vi "QCP_Load.vi"   [LabVIEW 2016]
uses:
  <userlib>/836-libraries/System/QCP_V2/QCPSupportCode/QCP_GetDbl.vi
  <userlib>/836-libraries/System/QCP_V2/QCPSupportCode/QCP_GetDblArr.vi
types:
  T1 = typedef "QCP_RefNum.ctl" = cluster{"Data Value Refnum":refnum<data-value>, "semaphore":T2}
  T2 = typedef "Semaphore RefNum" = refnum<k1>
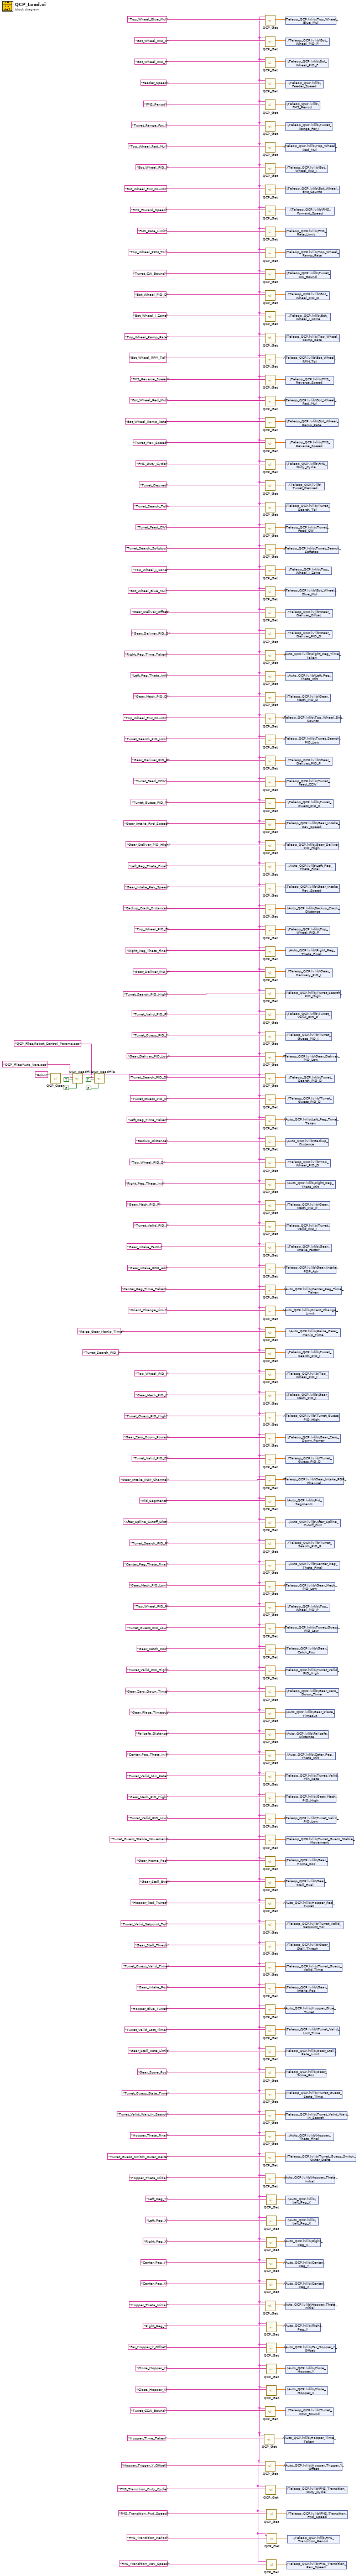
[diagram p0: block diagram]
diagram:
  n1 = call <userlib>:"QCP_Open.vi"("Name"="Robot") -> ("QCP_DevRef_Out"=w250:T1)  [unwired: 9 in, 1 out]
  n2 = call <userlib>:"QCP_ReadFile.vi"("Overrite Existing Data?"=FALSE ("Path Relative?"), "Path Relative?"=TRUE, "Path"="QCP_Files/Auto_Vars.qcp", "QCP_DevRef_In"=w250) -> ("QCP_DevRef_Out"=w245:T1)  [unwired: 6 in, 1 out]
  n3 = call <userlib>:"QCP_ReadFile.vi"("Overrite Existing Data?"=FALSE ("Path Relative?"), "Path Relative?"=TRUE, "Path"="QCP_Files/Robot_Control_Params.qcp", "QCP_DevRef_In"=w245) -> ("QCP_DevRef_Out"=w1:T1)  [unwired: 6 in, 1 out]
  n4 = call-poly <userlib>:"QCP_Get.vi"("Value Name"="Hopper_Time_Taken", "QCP_DevRef_In"=w1) -> ("Value"=w13:dbl)  [unwired: 7 in, 2 out]
  n5 = call-poly <userlib>:"QCP_Get.vi"("Value Name"="Top_Wheel_Blue_Mul", "QCP_DevRef_In"=w1) -> ("Value"=w75:dbl)  [unwired: 7 in, 2 out]
  n6 = call-poly <userlib>:"QCP_Get.vi"("Value Name"="Bot_Wheel_PID_P", "QCP_DevRef_In"=w1) -> ("Value"=w71:dbl)  [unwired: 7 in, 2 out]
  n7 = call-poly <userlib>:"QCP_Get.vi"("Value Name"="Bot_Wheel_PID_F", "QCP_DevRef_In"=w1) -> ("Value"=w70:dbl)  [unwired: 7 in, 2 out]
  n8 = call-poly <userlib>:"QCP_Get.vi"("Value Name"="Feeder_Speed", "QCP_DevRef_In"=w1) -> ("Value"=w102:dbl)  [unwired: 7 in, 2 out]
  n9 = call-poly <userlib>:"QCP_Get.vi"("Value Name"="FMS_Period", "QCP_DevRef_In"=w1) -> ("Value"=w25:dbl)  [unwired: 7 in, 2 out]
  n10 = call-poly <userlib>:"QCP_Get.vi"("Value Name"="Turret_Range_For_I", "QCP_DevRef_In"=w1) -> ("Value"=w17:dbl)  [unwired: 7 in, 2 out]
  n11 = call-poly <userlib>:"QCP_Get.vi"("Value Name"="Top_Wheel_Red_Mul", "QCP_DevRef_In"=w1) -> ("Value"=w76:dbl)  [unwired: 7 in, 2 out]
  n12 = call-poly <userlib>:"QCP_Get.vi"("Value Name"="Bot_Wheel_PID_I", "QCP_DevRef_In"=w1) -> ("Value"=w72:dbl)  [unwired: 7 in, 2 out]
  n13 = call-poly <userlib>:"QCP_Get.vi"("Value Name"="Bot_Wheel_Enc_Counts", "QCP_DevRef_In"=w1) -> ("Value"=w69:dbl)  [unwired: 7 in, 2 out]
  n14 = call-poly <userlib>:"QCP_Get.vi"("Value Name"="FMS_Foward_Speed", "QCP_DevRef_In"=w1) -> ("Value"=w101:dbl)  [unwired: 7 in, 2 out]
  n15 = call-poly <userlib>:"QCP_Get.vi"("Value Name"="FMS_Rate_Limit", "QCP_DevRef_In"=w1) -> ("Value"=w27:dbl)  [unwired: 7 in, 2 out]
  n16 = call-poly <userlib>:"QCP_Get.vi"("Value Name"="Top_Wheel_RPM_Tol", "QCP_DevRef_In"=w1) -> ("Value"=w77:dbl)  [unwired: 7 in, 2 out]
  n17 = call-poly <userlib>:"QCP_Get.vi"("Value Name"="Turret_CW_Bound", "QCP_DevRef_In"=w1) -> ("Value"=w24:dbl)  [unwired: 7 in, 2 out]
  n18 = call-poly <userlib>:"QCP_Get.vi"("Value Name"="Bot_Wheel_PID_D", "QCP_DevRef_In"=w1) -> ("Value"=w73:dbl)  [unwired: 7 in, 2 out]
  n19 = call-poly <userlib>:"QCP_Get.vi"("Value Name"="Bot_Wheel_I_Zone", "QCP_DevRef_In"=w1) -> ("Value"=w68:dbl)  [unwired: 7 in, 2 out]
  n20 = call-poly <userlib>:"QCP_Get.vi"("Value Name"="Top_Wheel_Ramp_Rate", "QCP_DevRef_In"=w1) -> ("Value"=w78:dbl)  [unwired: 7 in, 2 out]
  n21 = call-poly <userlib>:"QCP_Get.vi"("Value Name"="Bot_Wheel_RPM_Tol", "QCP_DevRef_In"=w1) -> ("Value"=w74:dbl)  [unwired: 7 in, 2 out]
  n22 = call-poly <userlib>:"QCP_Get.vi"("Value Name"="FMS_Reverse_Speed", "QCP_DevRef_In"=w1) -> ("Value"=w100:dbl)  [unwired: 7 in, 2 out]
  n23 = call-poly <userlib>:"QCP_Get.vi"("Value Name"="Bot_Wheel_Red_Mul", "QCP_DevRef_In"=w1) -> ("Value"=w66:dbl)  [unwired: 7 in, 2 out]
  n24 = call-poly <userlib>:"QCP_Get.vi"("Value Name"="Bot_Wheel_Ramp_Rate", "QCP_DevRef_In"=w1) -> ("Value"=w67:dbl)  [unwired: 7 in, 2 out]
  n25 = call-poly <userlib>:"QCP_Get.vi"("Value Name"="Turret_Max_Speed", "QCP_DevRef_In"=w1) -> ("Value"=w26:dbl)  [unwired: 7 in, 2 out]
  n26 = call-poly <userlib>:"QCP_Get.vi"("Value Name"="FMS_Duty_Cycle", "QCP_DevRef_In"=w1) -> ("Value"=w99:dbl)  [unwired: 7 in, 2 out]
  n27 = call-poly <userlib>:"QCP_Get.vi"("Value Name"="Turret_Desired", "QCP_DevRef_In"=w1) -> ("Value"=w21:dbl)  [unwired: 7 in, 2 out]
  n28 = call-poly <userlib>:"QCP_Get.vi"("Value Name"="Turret_Search_Tol", "QCP_DevRef_In"=w1) -> ("Value"=w22:dbl)  [unwired: 7 in, 2 out]
  n29 = call-poly <userlib>:"QCP_Get.vi"("Value Name"="Turret_Feed_CW", "QCP_DevRef_In"=w1) -> ("Value"=w20:dbl)  [unwired: 7 in, 2 out]
  n30 = call-poly <userlib>:"QCP_Get.vi"("Value Name"="Turret_Search_Softstop", "QCP_DevRef_In"=w1) -> ("Value"=w18:dbl)  [unwired: 7 in, 2 out]
  n31 = call-poly <userlib>:"QCP_Get.vi"("Value Name"="Top_Wheel_I_Zone", "QCP_DevRef_In"=w1) -> ("Value"=w81:dbl)  [unwired: 7 in, 2 out]
  n32 = call-poly <userlib>:"QCP_Get.vi"("Value Name"="Bot_Wheel_Blue_Mul", "QCP_DevRef_In"=w1) -> ("Value"=w79:dbl)  [unwired: 7 in, 2 out]
  n33 = call-poly <userlib>:"QCP_Get.vi"("Value Name"="Gear_Deliver_Offset", "QCP_DevRef_In"=w1) -> ("Value"=w51:dbl)  [unwired: 7 in, 2 out]
  n34 = call-poly <userlib>:"QCP_Get.vi"("Value Name"="Gear_Deliver_PID_D", "QCP_DevRef_In"=w1) -> ("Value"=w65:dbl)  [unwired: 7 in, 2 out]
  n35 = call-poly <userlib>:"QCP_Get.vi"("Value Name"="Right_Peg_Time_Taken", "QCP_DevRef_In"=w1) -> ("Value"=w129:dbl)  [unwired: 7 in, 2 out]
  n36 = call-poly <userlib>:"QCP_Get.vi"("Value Name"="Left_Peg_Theta_Init", "QCP_DevRef_In"=w1) -> ("Value"=w114:dbl)  [unwired: 7 in, 2 out]
  n37 = call-poly <userlib>:"QCP_Get.vi"("Value Name"="Gear_Mech_PID_D", "QCP_DevRef_In"=w1) -> ("Value"=w103:dbl)  [unwired: 7 in, 2 out]
  n38 = call-poly <userlib>:"QCP_Get.vi"("Value Name"="Top_Wheel_Enc_Counts", "QCP_DevRef_In"=w1) -> ("Value"=w82:dbl)  [unwired: 7 in, 2 out]
  n39 = call-poly <userlib>:"QCP_Get.vi"("Value Name"="Turret_Search_PID_Low", "QCP_DevRef_In"=w1) -> ("Value"=w30:dbl)  [unwired: 7 in, 2 out]
  n40 = call-poly <userlib>:"QCP_Get.vi"("Value Name"="Gear_Deliver_PID_P", "QCP_DevRef_In"=w1) -> ("Value"=w80:dbl)  [unwired: 7 in, 2 out]
  n41 = call-poly <userlib>:"QCP_Get.vi"("Value Name"="Turret_Feed_CCW", "QCP_DevRef_In"=w1) -> ("Value"=w29:dbl)  [unwired: 7 in, 2 out]
  n42 = call-poly <userlib>:"QCP_Get.vi"("Value Name"="Turret_Guess_PID_P", "QCP_DevRef_In"=w1) -> ("Value"=w31:dbl)  [unwired: 7 in, 2 out]
  n43 = call-poly <userlib>:"QCP_Get.vi"("Value Name"="Gear_Intake_Fwd_Speed", "QCP_DevRef_In"=w1) -> ("Value"=w52:dbl)  [unwired: 7 in, 2 out]
  n44 = call-poly <userlib>:"QCP_Get.vi"("Value Name"="Gear_Deliver_PID_High", "QCP_DevRef_In"=w1) -> ("Value"=w64:dbl)  [unwired: 7 in, 2 out]
  n45 = call-poly <userlib>:"QCP_Get.vi"("Value Name"="Left_Peg_Theta_Final", "QCP_DevRef_In"=w1) -> ("Value"=w113:dbl)  [unwired: 7 in, 2 out]
  n46 = call-poly <userlib>:"QCP_Get.vi"("Value Name"="Gear_Intake_Rev_Speed", "QCP_DevRef_In"=w1) -> ("Value"=w53:dbl)  [unwired: 7 in, 2 out]
  n47 = call-poly <userlib>:"QCP_Get.vi"("Value Name"="Backup_Crash_Distance", "QCP_DevRef_In"=w1) -> ("Value"=w104:dbl)  [unwired: 7 in, 2 out]
  n48 = call-poly <userlib>:"QCP_Get.vi"("Value Name"="Top_Wheel_PID_F", "QCP_DevRef_In"=w1) -> ("Value"=w83:dbl)  [unwired: 7 in, 2 out]
  n49 = call-poly <userlib>:"QCP_Get.vi"("Value Name"="Right_Peg_Theta_Final", "QCP_DevRef_In"=w1) -> ("Value"=w130:dbl)  [unwired: 7 in, 2 out]
  n50 = call-poly <userlib>:"QCP_Get.vi"("Value Name"="Gear_Deliver_PID_I", "QCP_DevRef_In"=w1) -> ("Value"=w84:dbl)  [unwired: 7 in, 2 out]
  n51 = call-poly <userlib>:"QCP_Get.vi"("Value Name"="Turret_Search_PID_High", "QCP_DevRef_In"=w1) -> ("Value"=w32:dbl)  [unwired: 7 in, 2 out]
  n52 = call-poly <userlib>:"QCP_Get.vi"("Value Name"="Turret_Valid_PID_P", "QCP_DevRef_In"=w1) -> ("Value"=w28:dbl)  [unwired: 7 in, 2 out]
  n53 = call-poly <userlib>:"QCP_Get.vi"("Value Name"="Turret_Guess_PID_I", "QCP_DevRef_In"=w1) -> ("Value"=w34:dbl)  [unwired: 7 in, 2 out]
  n54 = call-poly <userlib>:"QCP_Get.vi"("Value Name"="Gear_Deliver_PID_Low", "QCP_DevRef_In"=w1) -> ("Value"=w63:dbl)  [unwired: 7 in, 2 out]
  n55 = call-poly <userlib>:"QCP_Get.vi"("Value Name"="Turret_Search_PID_D", "QCP_DevRef_In"=w1) -> ("Value"=w33:dbl)  [unwired: 7 in, 2 out]
  n56 = call-poly <userlib>:"QCP_Get.vi"("Value Name"="Turret_Guess_PID_D", "QCP_DevRef_In"=w1) -> ("Value"=w35:dbl)  [unwired: 7 in, 2 out]
  n57 = call-poly <userlib>:"QCP_Get.vi"("Value Name"="Left_Peg_Time_Taken", "QCP_DevRef_In"=w1) -> ("Value"=w112:dbl)  [unwired: 7 in, 2 out]
  n58 = call-poly <userlib>:"QCP_Get.vi"("Value Name"="Backup_Distance", "QCP_DevRef_In"=w1) -> ("Value"=w105:dbl)  [unwired: 7 in, 2 out]
  n59 = call-poly <userlib>:"QCP_Get.vi"("Value Name"="Top_Wheel_PID_D", "QCP_DevRef_In"=w1) -> ("Value"=w86:dbl)  [unwired: 7 in, 2 out]
  n60 = call-poly <userlib>:"QCP_Get.vi"("Value Name"="Right_Peg_Theta_Init", "QCP_DevRef_In"=w1) -> ("Value"=w131:dbl)  [unwired: 7 in, 2 out]
  n61 = call-poly <userlib>:"QCP_Get.vi"("Value Name"="Gear_Mech_PID_P", "QCP_DevRef_In"=w1) -> ("Value"=w85:dbl)  [unwired: 7 in, 2 out]
  n62 = call-poly <userlib>:"QCP_Get.vi"("Value Name"="Turret_Valid_PID_I", "QCP_DevRef_In"=w1) -> ("Value"=w40:dbl)  [unwired: 7 in, 2 out]
  n63 = call-poly <userlib>:"QCP_Get.vi"("Value Name"="Gear_Intake_Factor", "QCP_DevRef_In"=w1) -> ("Value"=w54:dbl)  [unwired: 7 in, 2 out]
  n64 = call-poly <userlib>:"QCP_Get.vi"("Value Name"="Gear_Intake_PDP_Adr", "QCP_DevRef_In"=w1) -> ("Value"=w62:dbl)  [unwired: 7 in, 2 out]
  n65 = call-poly <userlib>:"QCP_Get.vi"("Value Name"="Center_Peg_Time_Taken", "QCP_DevRef_In"=w1) -> ("Value"=w132:dbl)  [unwired: 7 in, 2 out]
  n66 = call-poly <userlib>:"QCP_Get.vi"("Value Name"="Orient_Change_Limit", "QCP_DevRef_In"=w1) -> ("Value"=w111:dbl)  [unwired: 7 in, 2 out]
  n67 = call-poly <userlib>:"QCP_Get.vi"("Value Name"="Raise_Gear_Manip_Time", "QCP_DevRef_In"=w1) -> ("Value"=w106:dbl)  [unwired: 7 in, 2 out]
  n68 = call-poly <userlib>:"QCP_Get.vi"("Value Name"="Turret_Search_PID_I", "QCP_DevRef_In"=w1) -> ("Value"=w39:dbl)  [unwired: 7 in, 2 out]
  n69 = call-poly <userlib>:"QCP_Get.vi"("Value Name"="Top_Wheel_PID_I", "QCP_DevRef_In"=w1) -> ("Value"=w87:dbl)  [unwired: 7 in, 2 out]
  n70 = call-poly <userlib>:"QCP_Get.vi"("Value Name"="Gear_Mech_PID_I", "QCP_DevRef_In"=w1) -> ("Value"=w88:dbl)  [unwired: 7 in, 2 out]
  n71 = call-poly <userlib>:"QCP_Get.vi"("Value Name"="Turret_Guess_PID_High", "QCP_DevRef_In"=w1) -> ("Value"=w36:dbl)  [unwired: 7 in, 2 out]
  n72 = call-poly <userlib>:"QCP_Get.vi"("Value Name"="Gear_Zero_Down_Power", "QCP_DevRef_In"=w1) -> ("Value"=w55:dbl)  [unwired: 7 in, 2 out]
  n73 = call-poly <userlib>:"QCP_Get.vi"("Value Name"="Turret_Valid_PID_D", "QCP_DevRef_In"=w1) -> ("Value"=w41:dbl)  [unwired: 7 in, 2 out]
  n74 = call-poly <userlib>:"QCP_Get.vi"("Value Name"="Gear_Intake_PDP_Channel", "QCP_DevRef_In"=w1) -> ("Value"=w61:dbl)  [unwired: 7 in, 2 out]
  n75 = call-poly <userlib>:"QCP_Get.vi"("Value Name"="Pid_Segments", "QCP_DevRef_In"=w1) -> ("Value"=w110:dbl)  [unwired: 7 in, 2 out]
  n76 = call-poly <userlib>:"QCP_Get.vi"("Value Name"="After_Spline_Cutoff_Dist", "QCP_DevRef_In"=w1) -> ("Value"=w107:dbl)  [unwired: 7 in, 2 out]
  n77 = call-poly <userlib>:"QCP_Get.vi"("Value Name"="Turret_Search_PID_P", "QCP_DevRef_In"=w1) -> ("Value"=w19:dbl)  [unwired: 7 in, 2 out]
  n78 = call-poly <userlib>:"QCP_Get.vi"("Value Name"="Center_Peg_Theta_Final", "QCP_DevRef_In"=w1) -> ("Value"=w133:dbl)  [unwired: 7 in, 2 out]
  n79 = call-poly <userlib>:"QCP_Get.vi"("Value Name"="Gear_Mech_PID_Low", "QCP_DevRef_In"=w1) -> ("Value"=w91:dbl)  [unwired: 7 in, 2 out]
  n80 = call-poly <userlib>:"QCP_Get.vi"("Value Name"="Top_Wheel_PID_P", "QCP_DevRef_In"=w1) -> ("Value"=w89:dbl)  [unwired: 7 in, 2 out]
  n81 = call-poly <userlib>:"QCP_Get.vi"("Value Name"="Turret_Guess_PID_Low", "QCP_DevRef_In"=w1) -> ("Value"=w37:dbl)  [unwired: 7 in, 2 out]
  n82 = call-poly <userlib>:"QCP_Get.vi"("Value Name"="Gear_Catch_Pos", "QCP_DevRef_In"=w1) -> ("Value"=w56:dbl)  [unwired: 7 in, 2 out]
  n83 = call-poly <userlib>:"QCP_Get.vi"("Value Name"="Turret_Valid_PID_High", "QCP_DevRef_In"=w1) -> ("Value"=w42:dbl)  [unwired: 7 in, 2 out]
  n84 = call-poly <userlib>:"QCP_Get.vi"("Value Name"="Gear_Zero_Down_Time", "QCP_DevRef_In"=w1) -> ("Value"=w60:dbl)  [unwired: 7 in, 2 out]
  n85 = call-poly <userlib>:"QCP_Get.vi"("Value Name"="Gear_Place_Timeout", "QCP_DevRef_In"=w1) -> ("Value"=w109:dbl)  [unwired: 7 in, 2 out]
  n86 = call-poly <userlib>:"QCP_Get.vi"("Value Name"="Failsafe_Distance", "QCP_DevRef_In"=w1) -> ("Value"=w108:dbl)  [unwired: 7 in, 2 out]
  n87 = call-poly <userlib>:"QCP_Get.vi"("Value Name"="Center_Peg_Theta_Init", "QCP_DevRef_In"=w1) -> ("Value"=w134:dbl)  [unwired: 7 in, 2 out]
  n88 = call-poly <userlib>:"QCP_Get.vi"("Value Name"="Turret_Valid_Min_Rate", "QCP_DevRef_In"=w1) -> ("Value"=w44:dbl)  [unwired: 7 in, 2 out]
  n89 = call-poly <userlib>:"QCP_Get.vi"("Value Name"="Gear_Mech_PID_High", "QCP_DevRef_In"=w1) -> ("Value"=w90:dbl)  [unwired: 7 in, 2 out]
  n90 = call-poly <userlib>:"QCP_Get.vi"("Value Name"="Turret_Valid_PID_Low", "QCP_DevRef_In"=w1) -> ("Value"=w43:dbl)  [unwired: 7 in, 2 out]
  n91 = call-poly <userlib>:"QCP_Get.vi"("Value Name"="Turret_Guess_Stable_Movement", "QCP_DevRef_In"=w1) -> ("Value"=w38:dbl)  [unwired: 7 in, 2 out]
  n92 = call-poly <userlib>:"QCP_Get.vi"("Value Name"="Gear_Home_Pos", "QCP_DevRef_In"=w1) -> ("Value"=w57:dbl)  [unwired: 7 in, 2 out]
  n93 = call-poly <userlib>:"QCP_Get.vi"("Value Name"="Gear_Stall_Eval", "QCP_DevRef_In"=w1) -> ("Value"=w92:dbl)  [unwired: 7 in, 2 out]
  n94 = call-poly <userlib>:"QCP_Get.vi"("Value Name"="Hopper_Red_Turret", "QCP_DevRef_In"=w1) -> ("Value"=w128:dbl)  [unwired: 7 in, 2 out]
  n95 = call-poly <userlib>:"QCP_Get.vi"("Value Name"="Turret_Valid_Setpoint_Tol", "QCP_DevRef_In"=w1) -> ("Value"=w45:dbl)  [unwired: 7 in, 2 out]
  n96 = call-poly <userlib>:"QCP_Get.vi"("Value Name"="Gear_Stall_Thresh", "QCP_DevRef_In"=w1) -> ("Value"=w93:dbl)  [unwired: 7 in, 2 out]
  n97 = call-poly <userlib>:"QCP_Get.vi"("Value Name"="Turret_Guess_Valid_Time", "QCP_DevRef_In"=w1) -> ("Value"=w46:dbl)  [unwired: 7 in, 2 out]
  n98 = call-poly <userlib>:"QCP_Get.vi"("Value Name"="Gear_Intake_Pos", "QCP_DevRef_In"=w1) -> ("Value"=w58:dbl)  [unwired: 7 in, 2 out]
  n99 = call-poly <userlib>:"QCP_Get.vi"("Value Name"="Hopper_Blue_Turret", "QCP_DevRef_In"=w1) -> ("Value"=w127:dbl)  [unwired: 7 in, 2 out]
  n100 = call-poly <userlib>:"QCP_Get.vi"("Value Name"="Turret_Valid_Lost_Time", "QCP_DevRef_In"=w1) -> ("Value"=w47:dbl)  [unwired: 7 in, 2 out]
  n101 = call-poly <userlib>:"QCP_Get.vi"("Value Name"="Gear_Stall_Rate_Limit", "QCP_DevRef_In"=w1) -> ("Value"=w94:dbl)  [unwired: 7 in, 2 out]
  n102 = call-poly <userlib>:"QCP_Get.vi"("Value Name"="Gear_Score_Pos", "QCP_DevRef_In"=w1) -> ("Value"=w59:dbl)  [unwired: 7 in, 2 out]
  n103 = call-poly <userlib>:"QCP_Get.vi"("Value Name"="Turret_Guess_State_Time", "QCP_DevRef_In"=w1) -> ("Value"=w49:dbl)  [unwired: 7 in, 2 out]
  n104 = call-poly <userlib>:"QCP_Get.vi"("Value Name"="Turret_Valid_Wait_In_Search", "QCP_DevRef_In"=w1) -> ("Value"=w48:dbl)  [unwired: 7 in, 2 out]
  n105 = call-poly <userlib>:"QCP_Get.vi"("Value Name"="Hopper_Theta_Final", "QCP_DevRef_In"=w1) -> ("Value"=w126:dbl)  [unwired: 7 in, 2 out]
  n106 = call-poly <userlib>:"QCP_Get.vi"("Value Name"="Turret_Guess_Switch_Outer_Delta", "QCP_DevRef_In"=w1) -> ("Value"=w50:dbl)  [unwired: 7 in, 2 out]
  n107 = call-poly <userlib>:"QCP_Get.vi"("Value Name"="Hopper_Theta_Initial", "QCP_DevRef_In"=w1) -> ("Value"=w125:dbl)  [unwired: 7 in, 2 out]
  n108 = call-poly <userlib>:"QCP_Get.vi"("Value Name"="Hopper_Theta_Initial", "QCP_DevRef_In"=w1) -> ("Value"=w119:dbl)  [unwired: 7 in, 2 out]
  n109 = call-poly <userlib>:"QCP_Get.vi"("Value Name"="Turret_CCW_Bound", "QCP_DevRef_In"=w1) -> ("Value"=w23:dbl)  [unwired: 7 in, 2 out]
  n110 = call-poly <userlib>:"QCP_Get.vi"("Value Name"="Hopper_Trigger_Y_Offset", "QCP_DevRef_In"=w1) -> ("Values"=w10:dbl[])  [unwired: 7 in, 2 out]
  n111 = call-poly <userlib>:"QCP_Get.vi"("Value Name"="FMS_Transition_Duty_Cycle", "QCP_DevRef_In"=w1) -> ("Value"=w9:dbl)  [unwired: 7 in, 2 out]
  n112 = call-poly <userlib>:"QCP_Get.vi"("Value Name"="Left_Peg_Y", "QCP_DevRef_In"=w1) -> ("Values"=w124:dbl[])  [unwired: 7 in, 2 out]
  n113 = call-poly <userlib>:"QCP_Get.vi"("Value Name"="Left_Peg_X", "QCP_DevRef_In"=w1) -> ("Values"=w123:dbl[])  [unwired: 7 in, 2 out]
  n114 = call-poly <userlib>:"QCP_Get.vi"("Value Name"="Right_Peg_X", "QCP_DevRef_In"=w1) -> ("Values"=w122:dbl[])  [unwired: 7 in, 2 out]
  n115 = call-poly <userlib>:"QCP_Get.vi"("Value Name"="Center_Peg_Y", "QCP_DevRef_In"=w1) -> ("Values"=w121:dbl[])  [unwired: 7 in, 2 out]
  n116 = call-poly <userlib>:"QCP_Get.vi"("Value Name"="Center_Peg_X", "QCP_DevRef_In"=w1) -> ("Values"=w120:dbl[])  [unwired: 7 in, 2 out]
  n117 = call-poly <userlib>:"QCP_Get.vi"("Value Name"="Right_Peg_Y", "QCP_DevRef_In"=w1) -> ("Values"=w118:dbl[])  [unwired: 7 in, 2 out]
  n118 = call-poly <userlib>:"QCP_Get.vi"("Value Name"="Far_Hopper_Y_Offset", "QCP_DevRef_In"=w1) -> ("Values"=w117:dbl[])  [unwired: 7 in, 2 out]
  n119 = call-poly <userlib>:"QCP_Get.vi"("Value Name"="Close_Hopper_Y", "QCP_DevRef_In"=w1) -> ("Values"=w116:dbl[])  [unwired: 7 in, 2 out]
  n120 = call-poly <userlib>:"QCP_Get.vi"("Value Name"="Close_Hopper_X", "QCP_DevRef_In"=w1) -> ("Values"=w115:dbl[])  [unwired: 7 in, 2 out]
  n121 = call-poly <userlib>:"QCP_Get.vi"("Value Name"="FMS_Transition_Fwd_Speed", "QCP_DevRef_In"=w1) -> ("Value"=w6:dbl)  [unwired: 7 in, 2 out]
  n122 = call-poly <userlib>:"QCP_Get.vi"("Value Name"="FMS_Transition_Rev_Speed", "QCP_DevRef_In"=w1) -> ("Value"=w4:dbl)  [unwired: 7 in, 2 out]
  n123 = call-poly <userlib>:"QCP_Get.vi"("Value Name"="FMS_Transition_Period", "QCP_DevRef_In"=w1) -> ("Value"=w3:dbl)  [unwired: 7 in, 2 out]
  n124 = shared-variable ".\\Auto_QCP.lvlib\\Hopper_Time_Taken"(w13) -> ()  [unwired: 1 in, 1 out]
  n125 = shared-variable ".\\Teleop_QCP.lvlib\\Top_Wheel_Blue_Mul"(w75) -> ()  [unwired: 1 in, 1 out]
  n126 = shared-variable ".\\Teleop_QCP.lvlib\\Bot_Wheel_PID_P"(w71) -> ()  [unwired: 1 in, 1 out]
  n127 = shared-variable ".\\Teleop_QCP.lvlib\\Bot_Wheel_PID_F"(w70) -> ()  [unwired: 1 in, 1 out]
  n128 = shared-variable ".\\Teleop_QCP.lvlib\\Feeder_Speed"(w102) -> ()  [unwired: 1 in, 1 out]
  n129 = shared-variable ".\\Teleop_QCP.lvlib\\FMS_Period"(w25) -> ()  [unwired: 1 in, 1 out]
  n130 = shared-variable ".\\Teleop_QCP.lvlib\\Turret_Range_For_I"(w17) -> ()  [unwired: 1 in, 1 out]
  n131 = shared-variable ".\\Teleop_QCP.lvlib\\Top_Wheel_Red_Mul"(w76) -> ()  [unwired: 1 in, 1 out]
  n132 = shared-variable ".\\Teleop_QCP.lvlib\\Bot_Wheel_PID_I"(w72) -> ()  [unwired: 1 in, 1 out]
  n133 = shared-variable ".\\Teleop_QCP.lvlib\\Bot_Wheel_Enc_Counts"(w69) -> ()  [unwired: 1 in, 1 out]
  n134 = shared-variable ".\\Teleop_QCP.lvlib\\FMS_Forward_Speed"(w101) -> ()  [unwired: 1 in, 1 out]
  n135 = shared-variable ".\\Teleop_QCP.lvlib\\FMS_Rate_Limit"(w27) -> ()  [unwired: 1 in, 1 out]
  n136 = shared-variable ".\\Teleop_QCP.lvlib\\Top_Wheel_Ramp_Rate"(w77) -> ()  [unwired: 1 in, 1 out]
  n137 = shared-variable ".\\Teleop_QCP.lvlib\\Turret_CW_Bound"(w24) -> ()  [unwired: 1 in, 1 out]
  n138 = shared-variable ".\\Teleop_QCP.lvlib\\Bot_Wheel_PID_D"(w73) -> ()  [unwired: 1 in, 1 out]
  n139 = shared-variable ".\\Teleop_QCP.lvlib\\Bot_Wheel_I_Zone"(w68) -> ()  [unwired: 1 in, 1 out]
  n140 = shared-variable ".\\Teleop_QCP.lvlib\\Top_Wheel_Ramp_Rate"(w78) -> ()  [unwired: 1 in, 1 out]
  n141 = shared-variable ".\\Teleop_QCP.lvlib\\Bot_Wheel_RPM_Tol"(w74) -> ()  [unwired: 1 in, 1 out]
  n142 = shared-variable ".\\Teleop_QCP.lvlib\\FMS_Reverse_Speed"(w100) -> ()  [unwired: 1 in, 1 out]
  n143 = shared-variable ".\\Teleop_QCP.lvlib\\Bot_Wheel_Red_Mul"(w66) -> ()  [unwired: 1 in, 1 out]
  n144 = shared-variable ".\\Teleop_QCP.lvlib\\Bot_Wheel_Ramp_Rate"(w67) -> ()  [unwired: 1 in, 1 out]
  n145 = shared-variable ".\\Teleop_QCP.lvlib\\FMS_Reverse_Speed"(w26) -> ()  [unwired: 1 in, 1 out]
  n146 = shared-variable ".\\Teleop_QCP.lvlib\\FMS_Duty_Cycle"(w99) -> ()  [unwired: 1 in, 1 out]
  n147 = shared-variable ".\\Teleop_QCP.lvlib\\Turret_Desired"(w21) -> ()  [unwired: 1 in, 1 out]
  n148 = shared-variable ".\\Teleop_QCP.lvlib\\Turret_Search_Tol"(w22) -> ()  [unwired: 1 in, 1 out]
  n149 = shared-variable ".\\Teleop_QCP.lvlib\\Turret_Feed_CW"(w20) -> ()  [unwired: 1 in, 1 out]
  n150 = shared-variable ".\\Teleop_QCP.lvlib\\Turret_Search_Softstop"(w18) -> ()  [unwired: 1 in, 1 out]
  n151 = shared-variable ".\\Teleop_QCP.lvlib\\Top_Wheel_I_Zone"(w81) -> ()  [unwired: 1 in, 1 out]
  n152 = shared-variable ".\\Teleop_QCP.lvlib\\Bot_Wheel_Blue_Mul"(w79) -> ()  [unwired: 1 in, 1 out]
  n153 = shared-variable ".\\Teleop_QCP.lvlib\\Gear_Deliver_Offset"(w51) -> ()  [unwired: 1 in, 1 out]
  n154 = shared-variable ".\\Teleop_QCP.lvlib\\Gear_Deliver_PID_D"(w65) -> ()  [unwired: 1 in, 1 out]
  n155 = shared-variable ".\\Auto_QCP.lvlib\\Right_Peg_Time_Taken"(w129) -> ()  [unwired: 1 in, 1 out]
  n156 = shared-variable ".\\Auto_QCP.lvlib\\Left_Peg_Theta_Init"(w114) -> ()  [unwired: 1 in, 1 out]
  n157 = shared-variable ".\\Teleop_QCP.lvlib\\Gear_Mech_PID_D"(w103) -> ()  [unwired: 1 in, 1 out]
  n158 = shared-variable ".\\Teleop_QCP.lvlib\\Top_Wheel_Enc_Counts"(w82) -> ()  [unwired: 1 in, 1 out]
  n159 = shared-variable ".\\Teleop_QCP.lvlib\\Turret_Search_PID_Low"(w30) -> ()  [unwired: 1 in, 1 out]
  n160 = shared-variable ".\\Teleop_QCP.lvlib\\Gear_Deliver_PID_P"(w80) -> ()  [unwired: 1 in, 1 out]
  n161 = shared-variable ".\\Teleop_QCP.lvlib\\Turret_Feed_CCW"(w29) -> ()  [unwired: 1 in, 1 out]
  n162 = shared-variable ".\\Teleop_QCP.lvlib\\Turret_Guess_PID_P"(w31) -> ()  [unwired: 1 in, 1 out]
  n163 = shared-variable ".\\Teleop_QCP.lvlib\\Gear_Intake_Rev_Speed"(w52) -> ()  [unwired: 1 in, 1 out]
  n164 = shared-variable ".\\Teleop_QCP.lvlib\\Gear_Deliver_PID_High"(w64) -> ()  [unwired: 1 in, 1 out]
  n165 = shared-variable ".\\Auto_QCP.lvlib\\Left_Peg_Theta_Final"(w113) -> ()  [unwired: 1 in, 1 out]
  n166 = shared-variable ".\\Teleop_QCP.lvlib\\Gear_Intake_Rev_Speed"(w53) -> ()  [unwired: 1 in, 1 out]
  n167 = shared-variable ".\\Auto_QCP.lvlib\\Backup_Crash_Distance"(w104) -> ()  [unwired: 1 in, 1 out]
  n168 = shared-variable ".\\Teleop_QCP.lvlib\\Top_Wheel_PID_F"(w83) -> ()  [unwired: 1 in, 1 out]
  n169 = shared-variable ".\\Auto_QCP.lvlib\\Right_Peg_Theta_Final"(w130) -> ()  [unwired: 1 in, 1 out]
  n170 = shared-variable ".\\Teleop_QCP.lvlib\\Gear_Delivery_PID_I"(w84) -> ()  [unwired: 1 in, 1 out]
  n171 = shared-variable ".\\Teleop_QCP.lvlib\\Turret_Search_PID_High"(w32) -> ()  [unwired: 1 in, 1 out]
  n172 = shared-variable ".\\Teleop_QCP.lvlib\\Turret_Valid_PID_P"(w28) -> ()  [unwired: 1 in, 1 out]
  n173 = shared-variable ".\\Teleop_QCP.lvlib\\Turret_Guess_PID_I"(w34) -> ()  [unwired: 1 in, 1 out]
  n174 = shared-variable ".\\Teleop_QCP.lvlib\\Gear_Deliver_PID_Low"(w63) -> ()  [unwired: 1 in, 1 out]
  n175 = shared-variable ".\\Teleop_QCP.lvlib\\Turret_Search_PID_D"(w33) -> ()  [unwired: 1 in, 1 out]
  n176 = shared-variable ".\\Teleop_QCP.lvlib\\Turret_Guess_PID_D"(w35) -> ()  [unwired: 1 in, 1 out]
  n177 = shared-variable ".\\Auto_QCP.lvlib\\Left_Peg_Time_Taken"(w112) -> ()  [unwired: 1 in, 1 out]
  n178 = shared-variable ".\\Auto_QCP.lvlib\\Backup_Distance"(w105) -> ()  [unwired: 1 in, 1 out]
  n179 = shared-variable ".\\Teleop_QCP.lvlib\\Top_Wheel_PID_D"(w86) -> ()  [unwired: 1 in, 1 out]
  n180 = shared-variable ".\\Auto_QCP.lvlib\\Right_Peg_Thata_Init"(w131) -> ()  [unwired: 1 in, 1 out]
  n181 = shared-variable ".\\Teleop_QCP.lvlib\\Gear_Mech_PID_P"(w85) -> ()  [unwired: 1 in, 1 out]
  n182 = shared-variable ".\\Teleop_QCP.lvlib\\Turret_Valid_PID_I"(w40) -> ()  [unwired: 1 in, 1 out]
  n183 = shared-variable ".\\Teleop_QCP.lvlib\\Gear_Intake_Factor"(w54) -> ()  [unwired: 1 in, 1 out]
  n184 = shared-variable ".\\Teleop_QCP.lvlib\\Gear_Intake_PDP_Adr"(w62) -> ()  [unwired: 1 in, 1 out]
  n185 = shared-variable ".\\Auto_QCP.lvlib\\Center_Peg_Time_Taken"(w132) -> ()  [unwired: 1 in, 1 out]
  n186 = shared-variable ".\\Auto_QCP.lvlib\\Orient_Change_Limit"(w111) -> ()  [unwired: 1 in, 1 out]
  n187 = shared-variable ".\\Auto_QCP.lvlib\\Raise_Gear_Manip_Time"(w106) -> ()  [unwired: 1 in, 1 out]
  n188 = shared-variable ".\\Teleop_QCP.lvlib\\Turret_Search_PID_I"(w39) -> ()  [unwired: 1 in, 1 out]
  n189 = shared-variable ".\\Teleop_QCP.lvlib\\Top_Wheel_PID_I"(w87) -> ()  [unwired: 1 in, 1 out]
  n190 = shared-variable ".\\Teleop_QCP.lvlib\\Gear_Mech_PID_I"(w88) -> ()  [unwired: 1 in, 1 out]
  n191 = shared-variable ".\\Teleop_QCP.lvlib\\Turret_Guess_PID_High"(w36) -> ()  [unwired: 1 in, 1 out]
  n192 = shared-variable ".\\Teleop_QCP.lvlib\\Gear_Zero_Down_Power"(w55) -> ()  [unwired: 1 in, 1 out]
  n193 = shared-variable ".\\Teleop_QCP.lvlib\\Turret_Guess_PID_D"(w41) -> ()  [unwired: 1 in, 1 out]
  n194 = shared-variable ".\\Teleop_QCP.lvlib\\Gear_Intake_PDP_Channel"(w61) -> ()  [unwired: 1 in, 1 out]
  n195 = shared-variable ".\\Auto_QCP.lvlib\\Pid_Segments"(w110) -> ()  [unwired: 1 in, 1 out]
  n196 = shared-variable ".\\Auto_QCP.lvlib\\After_Spline_Cutoff_Dist"(w107) -> ()  [unwired: 1 in, 1 out]
  n197 = shared-variable ".\\Teleop_QCP.lvlib\\Turret_Search_PID_P"(w19) -> ()  [unwired: 1 in, 1 out]
  n198 = shared-variable ".\\Auto_QCP.lvlib\\Center_Peg_Theta_Final"(w133) -> ()  [unwired: 1 in, 1 out]
  n199 = shared-variable ".\\Teleop_QCP.lvlib\\Gear_Mech_PID_Low"(w91) -> ()  [unwired: 1 in, 1 out]
  n200 = shared-variable ".\\Teleop_QCP.lvlib\\Top_Wheel_PID_P"(w89) -> ()  [unwired: 1 in, 1 out]
  n201 = shared-variable ".\\Teleop_QCP.lvlib\\Turret_Guess_PID_Low"(w37) -> ()  [unwired: 1 in, 1 out]
  n202 = shared-variable ".\\Teleop_QCP.lvlib\\Gear_Catch_Pos"(w56) -> ()  [unwired: 1 in, 1 out]
  n203 = shared-variable ".\\Teleop_QCP.lvlib\\Turret_Valid_PID_High"(w42) -> ()  [unwired: 1 in, 1 out]
  n204 = shared-variable ".\\Teleop_QCP.lvlib\\Gear_Zero_Down_Time"(w60) -> ()  [unwired: 1 in, 1 out]
  n205 = shared-variable ".\\Auto_QCP.lvlib\\Gear_Place_Timeout"(w109) -> ()  [unwired: 1 in, 1 out]
  n206 = shared-variable ".\\Auto_QCP.lvlib\\Failsafe_Distance"(w108) -> ()  [unwired: 1 in, 1 out]
  n207 = shared-variable ".\\Auto_QCP.lvlib\\Ceter_Peg_Theta_Init"(w134) -> ()  [unwired: 1 in, 1 out]
  n208 = shared-variable ".\\Teleop_QCP.lvlib\\Turret_Valid_Min_Rate"(w44) -> ()  [unwired: 1 in, 1 out]
  n209 = shared-variable ".\\Teleop_QCP.lvlib\\Gear_Mech_PID_High"(w90) -> ()  [unwired: 1 in, 1 out]
  n210 = shared-variable ".\\Teleop_QCP.lvlib\\Turret_Valid_PID_Low"(w43) -> ()  [unwired: 1 in, 1 out]
  n211 = shared-variable ".\\Teleop_QCP.lvlib\\Turret_Guess_Stable_Movement"(w38) -> ()  [unwired: 1 in, 1 out]
  n212 = shared-variable ".\\Teleop_QCP.lvlib\\Gear_Home_Pos"(w57) -> ()  [unwired: 1 in, 1 out]
  n213 = shared-variable ".\\Teleop_QCP.lvlib\\Gear_Stall_Eval"(w92) -> ()  [unwired: 1 in, 1 out]
  n214 = shared-variable ".\\Auto_QCP.lvlib\\Hopper_Red_Turret"(w128) -> ()  [unwired: 1 in, 1 out]
  n215 = shared-variable ".\\Teleop_QCP.lvlib\\Turret_Valid_Setpoint_Tol"(w45) -> ()  [unwired: 1 in, 1 out]
  n216 = shared-variable ".\\Teleop_QCP.lvlib\\Gear_Stall_Thresh"(w93) -> ()  [unwired: 1 in, 1 out]
  n217 = shared-variable ".\\Teleop_QCP.lvlib\\Turret_Guess_Valid_Time"(w46) -> ()  [unwired: 1 in, 1 out]
  n218 = shared-variable ".\\Teleop_QCP.lvlib\\Gear_Intake_Pos"(w58) -> ()  [unwired: 1 in, 1 out]
  n219 = shared-variable ".\\Auto_QCP.lvlib\\Hopper_Blue_Turret"(w127) -> ()  [unwired: 1 in, 1 out]
  n220 = shared-variable ".\\Teleop_QCP.lvlib\\Turret_Valid_Lost_Time"(w47) -> ()  [unwired: 1 in, 1 out]
  n221 = shared-variable ".\\Teleop_QCP.lvlib\\Gear_Stall_Rate_Limit"(w94) -> ()  [unwired: 1 in, 1 out]
  n222 = shared-variable ".\\Teleop_QCP.lvlib\\Gear_Score_Pos"(w59) -> ()  [unwired: 1 in, 1 out]
  n223 = shared-variable ".\\Teleop_QCP.lvlib\\Turret_Guess_State_Time"(w49) -> ()  [unwired: 1 in, 1 out]
  n224 = shared-variable ".\\Teleop_QCP.lvlib\\Turret_Valid_Wait_In_Search"(w48) -> ()  [unwired: 1 in, 1 out]
  n225 = shared-variable ".\\Auto_QCP.lvlib\\Hopper_Theta_Final"(w126) -> ()  [unwired: 1 in, 1 out]
  n226 = shared-variable ".\\Teleop_QCP.lvlib\\Turret_Guess_Switch_Outer_Delta"(w50) -> ()  [unwired: 1 in, 1 out]
  n227 = shared-variable ".\\Auto_QCP.lvlib\\Hopper_Theta_Initial"(w125) -> ()  [unwired: 1 in, 1 out]
  n228 = shared-variable ".\\Auto_QCP.lvlib\\Left_Peg_Y"(w124) -> ()  [unwired: 1 in, 1 out]
  n229 = shared-variable ".\\Auto_QCP.lvlib\\Left_Peg_X"(w123) -> ()  [unwired: 1 in, 1 out]
  n230 = shared-variable ".\\Auto_QCP.lvlib\\Right_Peg_X"(w122) -> ()  [unwired: 1 in, 1 out]
  n231 = shared-variable ".\\Auto_QCP.lvlib\\Center_Peg_Y"(w121) -> ()  [unwired: 1 in, 1 out]
  n232 = shared-variable ".\\Auto_QCP.lvlib\\Center_Peg_X"(w120) -> ()  [unwired: 1 in, 1 out]
  n233 = shared-variable ".\\Auto_QCP.lvlib\\Hopper_Theta_Initial"(w119) -> ()  [unwired: 1 in, 1 out]
  n234 = shared-variable ".\\Auto_QCP.lvlib\\Right_Peg_Y"(w118) -> ()  [unwired: 1 in, 1 out]
  n235 = shared-variable ".\\Auto_QCP.lvlib\\Far_Hopper_Y_Offset"(w117) -> ()  [unwired: 1 in, 1 out]
  n236 = shared-variable ".\\Auto_QCP.lvlib\\Close_Hopper_Y"(w116) -> ()  [unwired: 1 in, 1 out]
  n237 = shared-variable ".\\Auto_QCP.lvlib\\Close_Hopper_X"(w115) -> ()  [unwired: 1 in, 1 out]
  n238 = shared-variable ".\\Teleop_QCP.lvlib\\Turret_CCW_Bound"(w23) -> ()  [unwired: 1 in, 1 out]
  n239 = shared-variable ".\\Auto_QCP.lvlib\\Hopper_Trigger_Y_Offset"(w10) -> ()  [unwired: 1 in, 1 out]
  n240 = shared-variable ".\\Teleop_QCP.lvlib\\FMS_Transition_Duty_Cycle"(w9) -> ()  [unwired: 1 in, 1 out]
  n241 = shared-variable ".\\Teleop_QCP.lvlib\\FMS_Transition_Fwd_Speed"(w6) -> ()  [unwired: 1 in, 1 out]
  n242 = shared-variable ".\\Teleop_QCP.lvlib\\FMS_Transition_Rev_Speed"(w4) -> ()  [unwired: 1 in, 1 out]
  n243 = shared-variable ".\\Teleop_QCP.lvlib\\FMS_Transition_Period"(w3) -> ()  [unwired: 1 in, 1 out]
